vi "AlliGator All ROIs Phasor Analysis.vi"(8 "error in (no error)":errorcluster, 10 "New Plot Name":string, 11 "AlliGator Internal Variables DVR":refnum<data-value>) -> (0 "error out":errorcluster, 1 "Calibrated Phasor":T1, 2 "Phasor Plot":cluster{"g Array":dbl[], "s Array":dbl[]}, 3 "AlliGator Internal Variables DVR":refnum<data-value>, 4 "Calibrated Phase Lifetime":dbl[unit], 6 "Message":string)   [LabVIEW 2021, in "AlliGator Phasor Graph.lvlib"]
doc: "Non-interactive phasor analysis of all ROIs."
uses:
  AlliGator Phasor Graph.lvlib
  AlliGator Internal Variables v2.ctl
  <vilib>/vision/Image Controls.llb/IMAQ Image.ctl
  AlliGator Gate Image Set.ctl
  AlliGator FLI Dataset Type.ctl
  AlliGator Data Series Type.ctl
  AlliGator Dataset Channel.ctl
  AlliGator Gate Arithmetic.ctl
  AlliGator Displayed Image.ctl
  Image/Named ROI Description.ctl
  AlliGator Decay Metadata v3.ctl
  AlliGator Decay Background Subtraction Info.ctl
  AlliGator Baseline Subtraction Method.ctl
  Graphs/XY Graph/XY Graph Plot Shift Parameters.ctl
  Graphs/XY Graph/XY Graph Plot Shift Method.ctl
  AlliGator Decay Extrapolation Parameters.ctl
  Phasor/Calibration Phasor (m, phi).ctl
  Phasor/Phasor Reference Series.ctl
  Phasor/Phasor Calibration Map v2.ctl
  Phasor/Phasor (g, s).ctl
  AlliGator Raw Phasor Plot Data v4.ctl
  Phasor/Phasor Standard Deviation Options.ctl
  AlliGator Phasor Multi-Harmonic Data.ctl
  Phasor/Phasor Harmonic Data.ctl
  AlliGator Decay Fit Options & Parameters v2.ctl
  Fits/IRF(X)PSED/Decay Fit Options v2.ctl
  Fits/Decay Convolution/Decay Model.ctl
  Fits/Residual Type.ctl
  Fits/IRF(X)PSED/Fit Weights Type.ctl
  Fits/Non-linear Fitting Method v2.ctl
  Fits/Fit Calculation Method.ctl
  Fits/Non-linear Fitting Algorithm.ctl
  AlliGator Decay Fit Parameter Constraints 2.ctl
  Fits/IRF(X)PSED/Decay Fit Parameters In List.ctl
  Fits/IRF(X)PSED/MLE Baseline Offset Type.ctl
  AlliGator Decay Preprocessing Parameters.ctl
  Fits/IRF(X)PSED/Decay Fit Parameters & Derived Quantities List.ctl
  AlliGator Variables List.ctl
  AlliGator Settings List.ctl
  Variant/Variant to Data/Variant to U16.vi
  <vilib>/Utility/error.llb/Error Cluster From Error Code.vi
  AlliGator Abort.vi
  <vilib>/ErrorRing/Error Ring.xnode
  AlliGator Globals, Variables & Constants.lvlib
  Image/Image.lvlib
  AlliGator Decay Processing.lvlib
  AlliGator Source Image.lvlib
  AlliGator Phasor Calibration.lvlib
  AlliGator Settings.lvlib
  Phasor/Phasor.lvlib
  Strings/Strings.lvlib
  Time/Time.lvlib
  AlliGator Decay Preprocessing.lvlib
  Graphs/XY Graph/XY Graph Add-Ons.lvlib
  GUI/GUI.lvlib
  Notebook/Notebook.lvlib
  Rich Text Box/Rich Text Box.lvlib
  Error/Error.lvlib
  Variant/Variant to Data/Variant to Data.lvlib
  AlliGator Files.lvlib
  AlliGator Internal Variables.lvlib
  AlliGator Phasor Plot.lvlib
  Fits/Fits.lvlib
  AlliGator Decay Fit.lvlib
  AlliGator Decay Fit Parameter Map.lvlib
  AlliGator Dual-Channel Datasets.lvlib
panel:
  # "see the AlliGator License on the block diagram (Ctrl+E or Window:Show Block Diagram)"
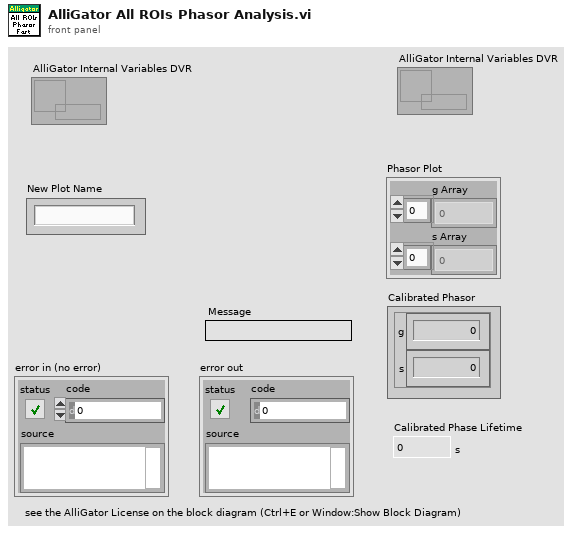
[diagram p1: front panel]
types:
  T1 = typedef "Phasor.lvlib/Phasor (g, s).ctl" = cluster{"g":dbl, "s":dbl}
  T2 = typedef "Phasor.lvlib/Phasor Standard Deviation Options.ctl" = cluster{"Compute Estimated SDV":bool, "# Replicas":u32, "Use Estimated Average Phasor":bool}
  T3 = typedef "AlliGator Settings.lvlib/AlliGator Settings List.ctl" = enum16{"GUI:Visible Settings Tab", "GUI:Last Run Version", "Source Image:Use Image Histogram for Contrast", "Source Image:Low Count Pixels Rejection Options", "Source Image:High Count Pixels Rejection Options", "Source Image:Use Image Brightness", "Source Image:Blend Overlay with Image Background", "Source Image:Use Fixed ROI Diameter", "Source Image:ROI Diameter", "Source Image:ROI Center Color", "Source Image:Peak Threshold", "Source Image:Intensity Threshold", "Source Image:Image Binning Options", "Source Image:Image Smoothing Options", "Source Image:Image Histogram Active", "Source Image:Invert Binary Mask", "Source Image:Hot Pixel Removal", "Source Image:Overlay Analyzed ROI Center", "Source Image:Auto-Adjust Contrast", "Source Image:Histogram Lower Percentile", "Source Image:Histogram Upper Percentile", "Source Image:Save Source Image", "Source Image:Scale Bar Options", "Source Image:Image Resolution (Pixel Size)", "Source Image:Flatfield Correction", "Source Image:Show Dead Left Columns Correction", "Source Image:Dead Left Columns Correction", "Source Image:Image Pre-Processing Operations Order", "Data Information:Gate Width", "Data Information:Nanotime Gate Separation", "Data Information:Macrotime Gate Separation", "Data Information:Gate Step", "Data Information:# Gates", "Data Information:Gate Image Exposure", "Data Information:Gate Image Integration", "Data Information:Gates to Skip", "Data Information:Gates to Keep", "Data Information:Define Gates to", "Data Information:Channel Name", "Data Information:Available Channel Names", "Data Information:Channel Arithmetic", "Data Information:Background File Subtraction", "Data Information:Background File", "Data Information:Background Scaling Factor", "Data Information:Background Pile-up Correction", "Data Information:Background Pixel Well Capacity", "Data Information:Laser Period", "Data Information:SYNC Period", "Data Information:Pile-up Correction", "Data Information:Pixel Well Capacity", "Data Information:Dataset Scaling Factor", "Fluorescence Decay_Decay Pre-Processing:Reverse Gates", "Fluorescence Decay_Decay Pre-Processing:Verbose Decay Pre-Processing", "Fluorescence Decay_Decay Pre-Processing:Use Decay Pre-Processing", "Fluorescence Decay_Decay Pre-Processing:Background Subtraction", "Fluorescence Decay_Decay Pre-Processing:Background Definition Range", "Fluorescence Decay_Decay Pre-Processing:Baseline Subtraction Method", "Fluorescence Decay_Decay Pre-Processing:Decay Pre-Processing Operations Order", "Fluorescence Decay_Decay Pre-Processing:Smoothing Parameter", "Fluorescence Decay_Decay Pre-Processing:Shift Decay", "Fluorescence Decay_Decay Pre-Processing:Decay Shift Parameters", "Fluorescence Decay_Decay Pre-Processing:Fold Decay", "Fluorescence Decay_Decay Pre-Processing:# Folds", "Fluorescence Decay_Decay Pre-Processing:1-Normalize Decay", "Fluorescence Decay_Decay Pre-Processing:[0-1]-Normalize Decay", "Fluorescence Decay_Decay Pre-Processing:Smoothen Decay", "Fluorescence Decay_Decay Pre-Processing:Extrapolate Decay", "Fluorescence Decay_Decay Pre-Processing:Use Periodicity", "Fluorescence Decay_Decay Pre-Processing:Use Cursors", "Fluorescence Decay_Decay Pre-Processing:Tail Fraction", "Fluorescence Decay_Decay Pre-Processing:Head Fraction", "Fluorescence Decay_Decay Pre-Processing:Additional Points", "Fluorescence Decay_Decay Pre-Processing:Straighten Decay", "Fluorescence Decay_Decay Pre-Processing:Constant Background", "Fluorescence Decay_Decay Pre-Processing:Pixel-Normalize Decay", "Fluorescence Decay_Advanced Analysis:Extract IRF instead of Decay", "Fluorescence Decay_Advanced Analysis:IRF Extraction Options", "Fluorescence Decay_Advanced Analysis:IRF Optimization Options", "Fluorescence Decay_Advanced Analysis:Square Pulse Options", "Fluorescence Decay_Advanced Analysis:IRF Order", "Fluorescence Decay_Advanced Analysis:IRF Time Constants", "Fluorescence Decay_Advanced Analysis:Wavelet Analysis Options", "Fluorescence Decay_Advanced Analysis:Average Lifetime Options", "Fluorescence Decay_Fit Options:Fit Options", "Fluorescence Decay_Fit Options:Use Legacy Fitting Approach", "Fluorescence Decay_Fit Options:Use Data Information Laser Period", "Fluorescence Decay_Fit Parameters:Displayed Fit Parameters", "Fluorescence Decay_Fit Parameters:Fit Parameter Constraints", "Fluorescence Decay_Fit Parameters:Export Tabulated Results", "Fluorescence Decay_Fit Parameters:MLE Baseline Offset Type", "Fluorescence Decay_Fit Parameters:MLE Baseline Offset", "Fluorescence Decay_Fit Parameters:Guess Parameter Names", "Fluorescence Decay_Fit Parameters:Guess Parameter Values", "Fluorescence Decay_Fit Parameters:Guess Parameters Options", "Fluorescence Decay_Styles:Show Last Decay Only", "Fluorescence Decay_Styles:Decay Graph Color Array", "Fluorescence Decay:Decay Graph Active", "Fluorescence Decay Statistics:Min Peak Value", "Fluorescence Decay Statistics:Reject Low Decay Peak Pixels", "Fluorescence Decay Statistics:Reject High Decay Peak Pixels", "Fluorescence Decay Statistics:Max Peak Value", "Time Traces:Use File Timestamp", "Time Traces:Time Step", "Time Traces:Use Intensity Correction File", "Time Traces:Intensity Correction File", "Phasor Plot:Phasor Plot Smoothing Options", "Phasor Plot:Phasor Plot Size", "Phasor Plot:Phasor Plot Graphics Options", "Phasor Plot:Cumulative Phasor Plot", "Phasor Plot:Use Phasor Brightness", "Phasor Plot:Blend Overlay with Phasor Background", "Phasor Plot:Save Phasor Plot", "Phasor Plot:Show References", "Phasor Plot:Phasor Ratio Decay Range", "Phasor Plot:Exponential Fading", "Phasor Plot:Phasor Ratio Reference Colors", "Phasor Plot:Reference Radius", "Phasor Plot:Show Color Map Vertices", "Phasor Plot:Phasor Plot Active", "Phasor Plot:Phasor Ratio Color Map Type", "Phasor Plot:Phasor Ratio Color Map", "Phasor Plot:Phasor Ratio Display Range", "Phasor Plot:Selected Image ROI(s)", "Phasor Plot:All Image ROIs", "Phasor Plot:Selected Phasor Plot ROI(s)", "Phasor Plot:All Phasor Plot ROIs", "Phasor Plot:Phasor Ratio Color-Coded Quantity", "Phasor Plot:Store Phasor Harmonics", "Phasor Plot:Draw Reference Segment", "Phasor Plot:User-Defined Quantity", "Phasor Graph:Phasor Frequency", "Phasor Graph:Phasor Ratio Type", "Phasor Graph:Pixel-level Phasor Computation", "Phasor Graph:Save Phasor Graph", "Phasor Graph:Phasor Graph Active", "Phasor Graph:Phasor SDV Options", "Phasor Calibration:Use Backup Calibration if needed", "Phasor Graph:Define Shortest Lifetime as", "Phasor Calibration:Backup Calibration Type", "Phasor Calibration:Calibration Type", "Phasor Calibration:Calibration Lifetime", "Phasor Calibration:Calibration Map Algorithm", "Single-Exponential Phasor Locus (SEPL):Gate Parameters", "Single-Exponential Phasor Locus (SEPL):User-defined Gate", "Single-Exponential Phasor Locus (SEPL):User-defined IRF", "Single-Exponential Phasor Locus (SEPL):Phasor Parameters", "Single-Exponential Phasor Locus (SEPL):Decay & IRF Parameters", "Single-Exponential Phasor Locus (SEPL):Display Parameters", "Lifetime Analysis:Decay Analysis Parameters", "Lifetime Analysis:Lifetime Map Active", "Plugins:Python Settings", "Miscellaneous:Verbose Mode", "Miscellaneous:Beep after Script", "Miscellaneous:Saved Image File Format", "Miscellaneous:Exported Gate Image Settings", "Miscellaneous:Include Loading in Timing", "Miscellaneous:Verbose Settings Mode", "Miscellaneous:Histogram Options", "Miscellaneous:Beep on Error", "Miscellaneous:# Logical Processors Used", "Miscellaneous:ROI Description Max Characters", "Miscellaneous:Verbose Error Mode", "Miscellaneous:Transparent Mask Color"}
  T4 = typedef "AlliGator Globals, Variables & Constants.lvlib/AlliGator Variables List.ctl" = enum16{"---- GUI ----", "Initialization Status", "State Indicators Refnum", "Original AlliGator Menu Items", "Current Action Loop State", "Script in progress", "Playback", "Loop Playback", "Search ROI Used", "Search ROI", "Decay Graph Max Legend Size", "Intensity Graph Max Legend Size", "Decay Statistics Graph Max Legend Size", "Phasor Graph Max Legend Size", "Phasor Ratio Graph Max Legend Size", "Lifetime Graph Max Legend Size", "---- Files ----", "Export Dataset Frames as Individual Files", "Show Batch Export Help Balloons", "Frames in Dataset", "ptu File Frame Start Indices", "Current Frame in Dataset", "Current Frame Timestamp", "------ Python Plugins ------", "Python Plugins Information", "Python Session", "Valid Python Session?", "---- Source Image ----", "Dataset Loaded", "Dataset Metadata", "Dataset Channel", "Dataset Data Description", "Background Dataset Metadata", "Background Dataset Channel", "Background Dataset Data Description", "Background File Subtraction", "Background File Path", "Background File Pile-up Correction", "Background File Pixel Well Capacity", "Background File Scaling Factor", "Source Image ROIs", "Current Source Image ROI", "Source Image ROI Event Refnum", "X_Source Image Display Range", "X_Source Image Palette Information", "Source Image Palette List", "Source Image Scale", "Current Dataset Load Settings", "Source Image:ROI Overlay Color", "---- Image Profile Window ----", "Image Profile:Overlay ROI in Source Image", "Image Profile Window Event Refnum", "Image Profile:IntensityType", "Image Profile:Intensity Average Type", "Image Profile:Intensity-weighted SDV", "Image Profile:Box Profile Type", "Image Profile Window Open", "Image Profile:Plotted Fit Parameter", "X_Type of Displayed Image", "X_Time Gate Slider", "Dataset Path", "Source Image Overlay to Erase", "Is Displayed Image Accumulated", "White Light Image Modified", "Mask Image Modified", "Macrotime Gate Separation", "------ Phasor Graph -------", "Phasor Graph:Show Line", "---- Phasor Plot ---", "Phasor Plot Parameters Changed", "FLI Dataset Modified since last Phasor Plot Calculation", "Phasor Harmonics Data", "Selected Phasor Harmonics", "Phasor Harmonic Manager Event Refnum", "Phasor Plot ROIs", "Current Phasor Plot ROI", "Phasor Plot ROI Event Refnum", "Phasor Plot Image Reference Points", "Phasor Plot Computed", "Phasor Plot Palette Information", "Phasor Plot Palette List", "Phasor Ratio Palette Information", "Phasor Ratio Palette List", "Phasor Image Scale", "Phasor Plot Image Overlay to Erase", "Phasor Plot Image Elements to Update", "Current Phasor Plot Calculation Parameters", "Current Phasor Calibration Options", "Reset Cumulated Phasor Plot", "Phasor Ratio Reference 1", "Phasor Ratio Lifetime Reference 1", "Phasor Ratio Reference 1 Frequency", "Phasor Ratio Reference 2", "Phasor Ratio Lifetime Reference 2", "Phasor Ratio Reference 2 Frequency", "---- Decay Analysis ----", "Number of Selected Decays to Fit", "LS Fit Results", "LAR Fit Results", "BS Fit Results", "Last Decay Max - Min", "Best Fit Parameters", "Best Fit Parameter Names", "Actual Size X", "Actual Size Y", "Binning X", "Binning Y", "Actual # Gates", "Dataset Number", "Gates to...", "Gates Skipped", "Gates to keep", "Gate Step", "Gate Separation", "Reversed Gates", "Pile-up Correction", "Pixel Well Capacity", "Background Subtracted", "Background Subtraction Method", "Background Definition Range", "Background File (deprecated)", "Number of Dataset Accumulated", "Array of Accumulated Dataset Paths", "Do Averaged Datasets", "Destination File Path", "Process Plot Target", "Use 1/D as Phasor Frequency", "---- Decay Fit Parameter Map -----", "Decay Fit Parameter Map Palette Information", "Decay Fit Parameter Map Palette List", "Local Decay Graph Window Event Refnum", "------- Local Decay Window ---------", "Use normalized IRF for convolution", "----- Miscellaneous ----", "Skippable Dialog Windows Status"}
  T5 = typedef "IMAQ Image.ctl" = refnum<image>
  T6 = typedef "Image.lvlib/Named ROI Description.ctl" = cluster{"ROI Descriptor":T7, "ROI Name":string, "Overlay Color":u32}
  T7 = typedef "ROI Descriptor" = cluster{"Global Rectangle":i32[], "Contours":cluster{"ID":enum32{"External", "Internal"}, "Type":u32, "Coordinates":i32[]}[]}
  T8 = typedef "AlliGator Phasor Graph.lvlib/AlliGator Raw Phasor Plot Data v4.ctl" = cluster{"Phasor Plot Name":string, "Raw Phasor Plot":T1[], "Phasor Frequency":dbl[unit], "[Decay Metadata]":T9[], "Raw Phasor Plot SDV":T1[], "Phasor SDV Options":T2, "[Calibration Phasor]":T15[]}
  T9 = typedef "AlliGator Phasor Graph.lvlib/AlliGator Decay Metadata v3.ctl" = cluster{"ROI Descriptor":T7, "ROI Center":cluster{"X":i32, "Y":i32}, "Decay Background Subtraction Info":T10, "Decay Reverted":bool, "Decay Smoothened":bool, "Decay Straightened":bool, "Fitted Tau (Decay Straightening)":dbl, "Decay Shift Parameters":T12, "Decay Shifted":bool, "Decay Extrapolated":bool, "Decay Extrapolation Parameters":T14, "Decay Normalized":bool, "Fold Decay":bool, "# Folds":u32}
  T10 = typedef "AlliGator Decay Analysis.lvlib/AlliGator Decay Preprocessing.lvlib/AlliGator Decay Background Subtraction Info.ctl" = cluster{"Laser Period":dbl[unit], "Gate Duration":dbl[unit], "Baseline Subtraction Method":T11, "Background Definition Range":cluster{"Min Gate":dbl[unit], "Max Gate":dbl[unit]}, "Total Intensity w/o Bkgd Subtraction":dbl, "Bkgd-subtracted Intensity (exp)":dbl, "# Data Points":i32, "Background/Gate":dbl, "Fitted Lifetime":dbl[unit], "Bkgd-subtracted Intensity (theo)":dbl}
  T11 = typedef "AlliGator Decay Analysis.lvlib/AlliGator Decay Preprocessing.lvlib/AlliGator Baseline Subtraction Method.ctl" = enum16{"Mean", "Min", "Square Gated Single-Exponential", "File", "Constant"}
  T12 = typedef "XY Graph Add-Ons.lvlib/XY Graph Plot Shift Parameters.ctl" = cluster{"Type":T13, "Shift":dbl[unit], "Threshold":dbl, "Rotate":bool}
  T13 = typedef "XY Graph Add-Ons.lvlib/XY Graph Plot Shift Method.ctl" = enum16{"Default", "CFD", "Threshold", "Cross-Correlation"}
  T14 = typedef "AlliGator Decay Analysis.lvlib/AlliGator Decay Preprocessing.lvlib/AlliGator Decay Extrapolation Parameters.ctl" = cluster{"Additional Points":u32, "Head Fraction":dbl, "Fitted Tau":dbl, "Use Periodicity":bool, "Use Cursors":bool, "Tail Fraction":dbl}
  T15 = typedef "Phasor.lvlib/Calibration Phasor (m, phi).ctl" = cluster{"m":dbl, "phi":dbl, "Phasor Frequency":dbl[unit], "Reference Lifetime":dbl[unit]}
  T16 = typedef "AlliGator Internal Variables.lvlib/AlliGator Internal Variables v2.ctl" = cluster{"Displayed Image":T5, "White Light Image":T5, "Mask Image":T5, "ROI Mask Image":T5, "Current Dataset Images 1":T17, "Background Dataset Images 1":T17, "Current Dataset Images 2":T17, "Background Dataset Images 2":T17, "Current Dataset Arithmetic Images":T17, "Accumulated Dataset Images 1":T17, "Accumulated Dataset Images 2":T17, "Accumulated Dataset Arithmetic Images":T17, "Phasor Plot Image":T5, "Decay Fit Parameter Map Image":T5, "Single Data Point Path":path, "White Light Image Path":path, "Mask Image Path":path, "Time-Series Folder":path, "[Time-Series Paths]":path[], "Current Dataset":i32, "Single Dataset Type":T18, "Current Folder":string, "AlliGator Data Series Type":T19, "# Datasets":i32, "Dual-Channel Dataset":bool, "Selected Channel Name":string, "Dataset Channel":T20, "Channel Arithmetic":T21, "Dual-Channel Background Dataset":bool, "Background Channel":T20, "Dual-Channel Accumulated Dataset":bool, "Start Time":dbl, "[Time-Series Timestamps]":dbl[], "[Intensity Corrections]":dbl[], "Time Series Script":bool, "Type of Displayed Image":T22, "Gate Image Slide":u16, "# Gates":i32, "ROIs":T6[], "ROI Decay":cluster{"t Array":dbl[], "I Array":dbl[]}, "Valid Decay":bool, "Decay  Metadata":T9, "Reference Decay Plot Name":string, "Reference Decay":cluster{"t Array":dbl[], "I Array":dbl[]}, "Decay Shift Plot":cluster{"Time Stamps":dbl[], "Decay Shifts":dbl[]}, "[Decays Max Values]":sgl[], "[Decays Min Values]":sgl[], "Calibration Phasor":T15, "Calibration Phasor Series":T23, "Phasor Calibration Map":T24, "Calibration Map MD5 Digest":string, "Last Raw Phasor":T1, "Last Calibrated Phasor":T1, "Last Calibrated Phasor SDV":T1, "Phasor Graph:Phasor Plot":cluster{"g Array":dbl[], "s Array":dbl[]}, "Phasor Graph:Phasor SDV Plot":cluster{"g Array":dbl[], "s Array":dbl[]}, "[Phasor Graph:Raw Phasor Plots]":T8[], "Phasor Plot locked to Ref 1":i32, "[Phasor Plot(s) locked to Ref 1]":i32[], "[Phasor Plot(s) locked to Ref 2]":i32[], "[Pixel Phasors]":T1[], "[[Sum Image]]":dbl[][], "[[CSG Phasors]]":csg[][], "[[Valid Pixel?]]":bool[][], "I/m/phi Dataset":cluster{"I/m/phi Dataset?":bool, "Base Frequency":dbl[unit], "Harmonic Orders":u8[]}, "Multi Phasor Plot Data":T25, "Decay Fit Options & Parameters":T27, "Fit Options: Decay Preprocessing Parameters":T38, "Fit Options: Reference Decay":cluster{"t Array":dbl[], "I Array":dbl[]}, "Is Full Image Parameters Map":bool, "Is Single-Pixels Parameters Map":bool, "NLSF Parameters Map X Resolution":i32, "NLSF Parameters Map Y Resolution":i32, "[Single Decay Fit Parameters]":dbl[], "Fit Model":T29, "[[Multiple Decays Fit Parameters]]":dbl[][], "[[Multiple Decays Fit Parameter SDVs]]":dbl[][], "[[IRFs]]":dbl[][], "IRF Array Time Axis":dbl[], "Decay Array Time Axis":dbl[], "[Decay Fit Parameter Names]":T39[], "[[Phasor Ratios]]":dbl[][], "[[Average Lifetimes]]":dbl[][], "Amplitude Weighted Average Lifetime":bool, "[Decay Sum]":dbl[], "[[User-defined Quantities]]":dbl[][], "User-defined Quantity":string}
  T17 = typedef "AlliGator Internal Variables.lvlib/AlliGator Gate Image Set.ctl" = cluster{"SGL Image Max":T5, "SGL Image Sum":T5, "SGL Gate Images":T5[], "SGL Image Min":T5}
  T18 = typedef "AlliGator Files.lvlib/AlliGator FLI Dataset Type.ctl" = enum16{"HDF5 FLI Dataset", "Gate Image Folder", ".sdt FLI Dataset (Becker & Hickl)", ".ptu FLI Dataset (PicoQuant)", "SS1 FLI Dataset", "SS2 FLI Dataset", "I/m/phi Dataset", ".bin FLI Dataset (PicoQuant Binned)", ".bin FLI Dataset (Piccolo Binned)"}
  T19 = typedef "AlliGator Files.lvlib/AlliGator Data Series Type.ctl" = enum16{"Not a Supported Series", "Gate Images Folder Series", "SwissSPAD 2 Dataset Series", "B&H FLI Dataset Series", "PicoQuant PTU FLI Dataset Series", "PicoQuant BIN FLI Dataset Series", "Piccolo hist BIN FLI Dataset Series", "HDF5 FLI Dataset Series"}
  T20 = typedef "AlliGator Dual-Channel Datasets.lvlib/AlliGator Dataset Channel.ctl" = enum16{"G2", "INT"}
  T21 = typedef "AlliGator Settings.lvlib/AlliGator Gate Arithmetic.ctl" = enum16{"None", "INT-G2", "G2/INT*<INT>", "(1 - G2/INT)*<INT>"}
  T22 = typedef "AlliGator Source Image.lvlib/AlliGator Displayed Image.ctl" = enum16{"Single Gate", "Sum of All Gates", "Max of All Gates", "Min of All Gates", "-", "White Ligth Image", "Mask Image"}
  T23 = typedef "Phasor.lvlib/Phasor Reference Series.ctl" = cluster{"m Array":dbl[], "phi Array":dbl[], "Phasor Frequency":dbl[unit], "Calibration Lifetime":dbl[unit]}
  T24 = typedef "Phasor.lvlib/Phasor Calibration Map v2.ctl" = cluster{"Phasor Frequency":dbl[unit], "Calibration Lifetime":dbl[unit], "ROI Centers":cluster{"X":i32, "Y":i32}[], "ROI Descriptors":T7[], "Map Resolution X":i32, "Map Resolution Y":i32, "z Array":cdb[]}
  T25 = typedef "AlliGator Phasor Plot.lvlib/AlliGator Phasor Multi-Harmonic Data.ctl" = cluster{"Base Frequency":dbl[unit], "# Harmonics":u8, "Harmonic Orders":u8[], "Phasor Plot Settings Checksum":u64, "Phasor Harmonic Data Array":T26[]}
  T26 = typedef "Phasor.lvlib/Phasor Harmonic Data.ctl" = cluster{"Phasor Harmonic Name":string, "Phasor Plot Settings Checksum":u64, "Phasor Frequency":dbl[unit], "Base Frequency":dbl[unit], "Harmonic Order":u8, "Phasor Plot Parameters":string, "Phasor Array [[CSG]]":csg[][], "Dataset File Path":path}
  T27 = typedef "AlliGator Decay Fit Parameter Map.lvlib/AlliGator Decay Fit Options & Parameters v2.ctl" = cluster{"SYNC Period":dbl[unit], "Fit Options":T28, "Fit Parameter Constraints":T35[], "MLE Baseline Offset":dbl, "MLE Baseline Offset Type":T37}
  T28 = typedef "Fits.lvlib/Decay Fit Options v2.ctl" = cluster{"Show Fit Residuals":bool, "Fit Model":T29, "Residual Type":T30, "Max Decay Percentile":dbl, "Min Decay Percentile":dbl, "Show Full Decay":bool, "Weights":T31, "Fitting Method":T32, "Compute Parameter Uncertainties":bool, "Periodic Boundaries":bool, "Model Calculation":T33, "Period":dbl[unit], "Termination Criteria":cluster{"Max Iterations":i32, "Max Function Calls":i32, "Max Time":dbl[unit], "Function Tolerance":dbl, "Parameter Tolerance":dbl, "Gradient Tolerance":dbl, "Min Lambda":dbl, "Max Lambda":dbl, "Initial Tick Count":u32}, "Offset Resolution":dbl[unit], "Use Local IRF":bool, "Fitting Algorithm":T34}
  T29 = typedef "Fits.lvlib/Decay Model.ctl" = enum16{"1-Exponential", "2-Exponentials"}
  T30 = typedef "Fits.lvlib/Residual Type.ctl" = enum16{"Standard", "Normalized", "Reduced"}
  T31 = typedef "Fits.lvlib/Fit Weights Type.ctl" = enum16{"Unweighted", "1/Variance", "Best of All"}
  T32 = typedef "Fits.lvlib/Non-linear Fitting Method v2.ctl" = enum16{"Least Square", "Least Absolute Residual", "Bisquare", "MLE", "-", "Best of All"}
  T33 = typedef "Fits.lvlib/Fit Calculation Method.ctl" = enum16{"Simulation", "Convolution", "Integration"}
  T34 = typedef "Fits.lvlib/Non-linear Fitting Algorithm.ctl" = enum16{"Levenberg-Marquardt", "Trust-Region Dogleg"}
  T35 = typedef "AlliGator Decay Analysis.lvlib/AlliGator Decay Fit.lvlib/AlliGator Decay Fit Parameter Constraints 2.ctl" = cluster{"Fit Parameter":T36, "Min Value":dbl, "Max Value":dbl, "Global":bool, "Used":bool}
  T36 = typedef "Fits.lvlib/Decay Fit Parameters In List.ctl" = enum16{"Offset", "Baseline", "A_1", "tau_1", "A_2", "tau_2"}
  T37 = typedef "Fits.lvlib/MLE Baseline Offset Type.ctl" = enum32{"Absolute", "Percentage"}
  T38 = typedef "AlliGator Decay Analysis.lvlib/AlliGator Decay Preprocessing.lvlib/AlliGator Decay Preprocessing Parameters.ctl" = cluster{"Background Subtraction":bool, "Straighten Decay":bool, "Reverse Gates":bool, "1-Normalized Decay":bool, "Smoothen Decay":bool, "Smoothing Parameter":dbl, "Shift Decay":bool, "Decay Shift Parameters":T12, "Extrapolate Decay":bool, "Additional Points":u32, "Head Fraction":dbl, "Pixel-Normalize Decay":bool, "Use Periodicity":bool, "Use Cursors":bool, "Tail Fraction":dbl, "Use Decay Pre-Processing":bool, "Fold Decay":bool, "# Folds":u32, "[0-1]-Normalized Decay":bool}
  T39 = typedef "Fits.lvlib/Decay Fit Parameters & Derived Quantities List.ctl" = enum16{"Offset", "Baseline", "A_1", "tau_1", "A_2", "tau_2", "<tau>_a", "f1_a", "f2_a", "<tau>_i", "f1_i", "f2_i", "-", "R^2", "Chi^2"}
  T40 = cluster{"Decay Peak Constraint":bool, "Min":dbl, "Max":dbl}
  T41 = typedef "AlliGator Settings.lvlib/AlliGator Pixel Counts Constraints.ctl" = cluster{"High Count Pixels Rejection Options":T42, "Low Count Pixels Rejection Options":T43}
  T42 = typedef "AlliGator Settings.lvlib/AlliGator High Count Pixels Rejection Options.ctl" = cluster{"Background High Threshold Factor":dbl, "Fixed High Background Threshold":dbl, "Reject High Count Pixels":bool, "High Percentile":dbl}
  T43 = typedef "AlliGator Settings.lvlib/AlliGator Low Count Pixels Rejection Options.ctl" = cluster{"Background Low Threshold Factor":dbl, "Fixed Low Background Threshold":dbl, "Reject Low Count Pixels":bool, "Low Percentile":dbl}
  T44 = cluster{"t Axis":dbl[], "ROI Intensity Array":dbl[]}
  T45 = typedef "Rich Text Box.lvlib/Text Formatting.ctl" = cluster{"Font":string, "Text Color":T46, "Text Background Color":T46, "Text Style":enum16{"Regular", "Bold", "Italic", "Underline", "Strikeout"}, "Font Size (Points)":dbl, "Text Alignment":i32}
  T46 = typedef "Rich Text Box.lvlib/Text Colors.ctl" = enum16{"Unchanged", "Black", "Blue", "Brown", "Gray", "Green", "Orange", "Pink", "Red", "White"}
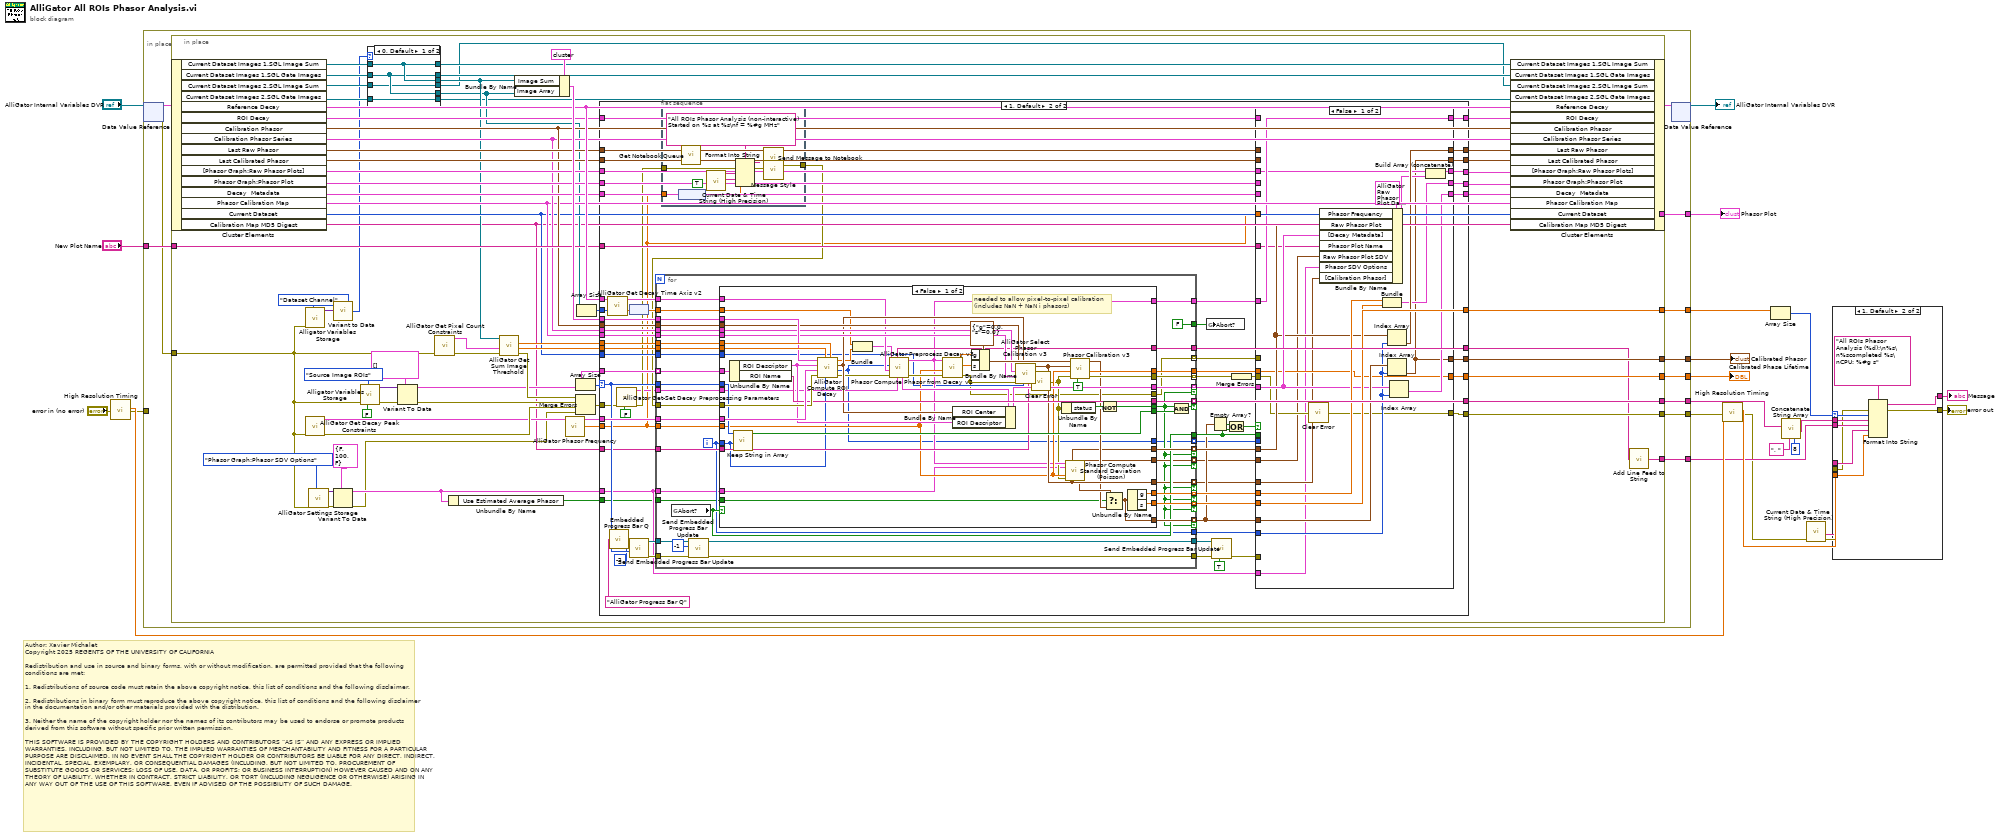
[diagram p0: block diagram]
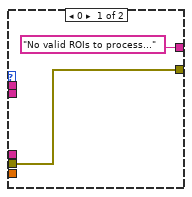
[diagram p2: hidden frame]
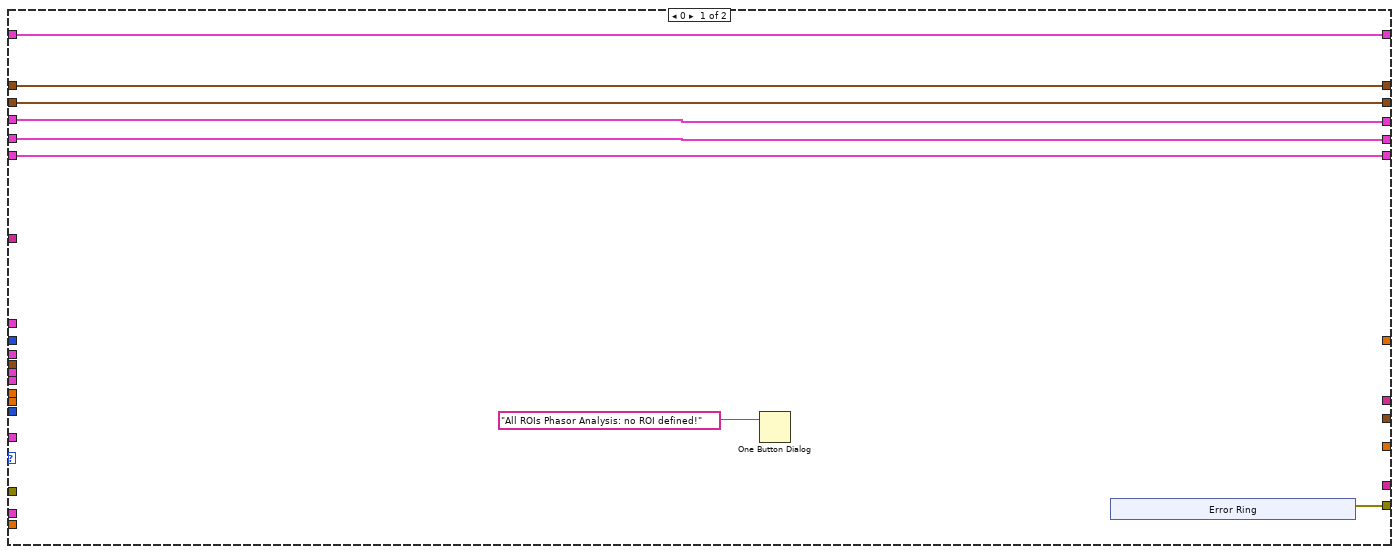
[diagram p4: hidden frame]
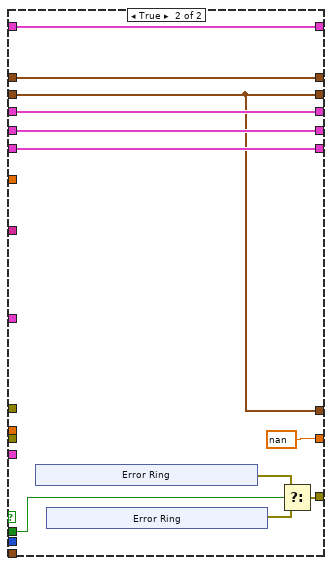
[diagram p5: hidden frame]
diagram:
  # "Author: Xavier Michalet\nCopyright 2025 REGENTS OF THE UNIVERSITY OF CALIFORNIA\n\nRedistribution and use in source and binary forms, with or without modification, are permitted provided that the following conditions are met:\n\n1. Redistributions of source code must retain the above copyright notice, this list of conditions and the following disclaimer.\n\n2. Redistributions in binary form must reproduce the above copyright notice, this list of conditions and the following disclaimer in the documentation and/or other materials provided with the distribution.\n\n3. Neither the name of the copyright holder nor the names of its contributors may be used to endorse or promote products derived from this software without specific prior written permission.\n\nTHIS SOFTWARE IS PROVIDED BY THE COPYRIGHT HOLDERS AND CONTRIBUTORS “AS IS” AND ANY EXPRESS OR IMPLIED WARRANTIES, INCLUDING, BUT NOT LIMITED TO, THE IMPLIED WARRANTIES OF MERCHANTABILITY AND FITNESS FOR A PARTICULAR PURPOSE ARE DISCLAIMED. IN NO EVENT SHALL THE COPYRIGHT HOLDER OR CONTRIBUTORS BE LIABLE FOR ANY DIRECT, INDIRECT, INCIDENTAL, SPECIAL, EXEMPLARY, OR CONSEQUENTIAL DAMAGES (INCLUDING, BUT NOT LIMITED TO, PROCUREMENT OF SUBSTITUTE GOODS OR SERVICES; LOSS OF USE, DATA, OR PROFITS; OR BUSINESS INTERRUPTION) HOWEVER CAUSED AND ON ANY THEORY OF LIABILITY, WHETHER IN CONTRACT, STRICT LIABILITY, OR TORT (INCLUDING NEGLIGENCE OR OTHERWISE) ARISING IN ANY WAY OUT OF THE USE OF THIS SOFTWARE, EVEN IF ADVISED OF THE POSSIBILITY OF SUCH DAMAGE."
  n1 = call "High Resolution Timing.vi"("Error In"="error in (no error)") -> ("elapsed (relative) seconds"=w13:dbl, "Error Out"=w7:errorcluster)  [unwired: 16 in, 1 out]
  n2 = in-place {
    in-place-border: [w32] -> w4
    in-place-border: [w31] -> w20
    in-place-border: "New Plot Name" -> [w30]
    in-place-border: [w29] -> w18
    in-place-border: [w28] -> w17
    in-place-border: [w27] -> w9
    in-place-border: w7 -> [_]
    in-place-border: [w25] -> w6
    in-place-border: [w24] -> w3
    n3 = in-place-dvr #1("AlliGator Internal Variables DVR") -> (w34:T16, w26:errorcluster)
    n4 = in-place {
      in-place-border: w26 -> [w43]
      in-place-border: [w85] -> w32
      in-place-border: [w73] -> w31
      in-place-border: w30 -> [w72]
      in-place-border: [w71] -> w29
      in-place-border: [w70] -> w28
      in-place-border: [w69] -> w27
      in-place-border: [w67] -> w25
      in-place-border: [w59] -> w24
      n5 = in-place-cluster #2(w34) -> ("Current Dataset Images 1.SGL Image Sum"=w53:T5, "Current Dataset Images 1.SGL Gate Images"=w52:T5[], "Current Dataset Images 2.SGL Image Sum"=w56:T5, "Current Dataset Images 2.SGL Gate Images"=w55:T5[], "Reference Decay"=w86:cluster{"t Array":dbl[], "I Array":dbl[]}, "ROI Decay"=w75:cluster{"t Array":dbl[], "I Array":dbl[]}, "Calibration Phasor"=w66:T15, "Calibration Phasor Series"=w65:T23, "Last Raw Phasor"=w84:T1, "Last Calibrated Phasor"=w82:T1, "[Phasor Graph:Raw Phasor Plots]"=w80:T8[], "Phasor Graph:Phasor Plot"=w78:cluster{"g Array":dbl[], "s Array":dbl[]}, "Decay  Metadata"=w77:T9, "Phasor Calibration Map"=w64:T24, "Current Dataset"=w62:i32, "Calibration Map MD5 Digest"=w51:string)
      n6 = call "Alligator Variables Storage.vi"("AlliGator Variable"=AlliGator_Variables_List."Dataset Channel" ("Alligator Variable"), "Error In"=w43) -> ("Data out"=w49:variant)  [unwired: 7 in, 2 out]
      n7 = call "AlliGator Get Decay Peak Constraints.vi"("error in (no error)"=w43) -> ("Error Out"=w90:errorcluster, "Decay Peak Constraints"=w89:T40)  [unwired: 9 in]
      n8 = call "AlliGator Settings Storage.vi"("AlliGator Settings List"=AlliGator_Settings_List."Phasor Graph:Phasor SDV Options", "Error In"=w43) -> ("Error Out"=w47:errorcluster, "Variant Data out"=w46:variant)  [unwired: 8 in]
      n9 = call-poly "Variant to Data.vi"("Variant"=w49) -> ("U16 Value"=w48:u16)  [unwired: 8 in]
      n10 = Variant To Data(error in=w47, type=T2 {"Compute Estimated SDV"=FALSE, "# Replicas"=100, "Use Estimated Average Phasor"=FALSE} ("Phasor SDV Options"), Variant=w46) -> (data=w36:T2, error out=w35:errorcluster)
      n11 = call "Alligator Variables Storage.vi"("Get(F)/Set"=FALSE, "AlliGator Variable"=AlliGator_Variables_List."Source Image ROIs" ("Alligator Variable"), "Error In"=w43) -> ("Error Out"=w99:errorcluster, "Data out"=w100:variant)  [unwired: 6 in, 1 out]
      n12 = case shown="0, Default" w48 {
        tunnel: [w105 w107] -> w57
        tunnel: w56 -> [w103 w107]
        tunnel: [w104 w106] -> w54
        tunnel: w55 -> [w102 w106]
        tunnel: w53 -> [w105 w109]
        tunnel: w52 -> [w104 w108]
        tunnel: [w105 w109] -> w41
        tunnel: [w104 w108] -> w40
        tunnel: [w103 w107] -> w39
        tunnel: [w102 w106] -> w38
        frame 0, Default {
        }
        frame 1 {
        }
      }
      n13 = Variant To Data(error in=w99, type=T6[] [] ("Stored ROIs in"), Variant=w100) -> (data=w61:T6[], error out=w94:errorcluster)
      n14 = call "AlliGator Get Pixel Count Constraints.vi"("error in (no error)"=w43) -> ("error out"=w95:errorcluster, "Pixel Count Constraints"=w96:T41)  [unwired: 9 in]
      n15 = Unbundle By Name(w36) -> ("Use Estimated Average Phasor"=w37:bool)
      n16 = call "AlliGator Get Sum Image Threshold.vi"("error in (no error)"=w95, "Pixel Counts Constraints"=w96, "Image in"=w57) -> ("error out"=w63:errorcluster, "Pixel Threshold Low"=w91:sgl, "Pixel Threshold High"=w92:sgl)  [unwired: 2 in, 4 out]
      n17 = Bundle By Name(cluster=cluster{"Image Sum":T5, "Image Array":T5[]} {"Image Sum"=refnum, "Image Array"=[]} ("Images"), "Image Sum"=w57, "Image Array"=w54) -> (w88:cluster{"Image Sum":T5, "Image Array":T5[]})
      n18 = call "AlliGator Phasor Frequency.vi"() -> ("Phasor Frequency"=w42:dbl[unit])
      n19 = Array Size(array=w61) -> (size(s)=w60:i32)
      n20 = Merge Errors(w63, w94, w90, w35) -> (w93:errorcluster)
      n21 = Array Size(array=w54) -> (size(s)=w87:i32)
      n22 = case shown="1, Default" w60 {
        selector: w60 -> [_ w145]
        tunnel: w93 -> [_ w140]
        tunnel: w92 -> [_ w189]
        tunnel: w91 -> [_ w188]
        tunnel: w89 -> [_ w187]
        tunnel: w88 -> [_ w186]
        tunnel: w87 -> [_ w185]
        tunnel: w86 -> [_ w183]
        tunnel: [w110 w182] -> w85
        tunnel: w84 -> [w116 w181]
        tunnel: [w116 w180] -> w83
        tunnel: w82 -> [w115 w179]
        tunnel: [w115 w178] -> w81
        tunnel: w80 -> [w114 w177]
        tunnel: [w114 w176] -> w79
        tunnel: w78 -> [w113 w175]
        tunnel: w77 -> [w112 w173]
        tunnel: [w112 w172] -> w76
        tunnel: w75 -> [w117 w169]
        tunnel: [w117 w168] -> w74
        tunnel: w42 -> [_ w125]
        tunnel: [_ w165] -> w73
        tunnel: w72 -> [_ w164]
        tunnel: [w113 w163] -> w71
        tunnel: [_ w162] -> w70
        tunnel: [_ w159] -> w69
        tunnel: [_ w157] -> w68
        tunnel: w66 -> [_ w156]
        tunnel: w65 -> [_ w155]
        tunnel: w64 -> [_ w154]
        tunnel: w62 -> [_ w152]
        tunnel: w61 -> [_ w150]
        tunnel: [_ w143] -> w59
        tunnel: w51 -> [_ w129]
        tunnel: w36 -> [_ w126]
        tunnel: w37 -> [_ w124]
        frame 0 {
          n23 = One Button Dialog(message="All ROIs Phasor Analysis: no ROI defined!") -> ()  [unwired: 1 in, 1 out]
          n24 = xnode "Error Ring"() -> ("error out"=w110:errorcluster)
        }
        frame 1, Default {
          n25 = call "AlliGator Get Decay Time Axis v2.vi"("Number of Gates"=w185) -> ("t Array"=w184:dbl[unit][])  [unwired: 14 in]
          n26 = call "Embedded Progress Bar Q.vi"("Progress Bar Queue Name"="AlliGator Progress Bar Q") -> ("Progress Bar Queue"=w132:refnum<queue>)  [unwired: 6 in]
          n27 = call "AlliGator Get-Set Decay Preprocessing Parameters.vi"("Get (F)/Set"=FALSE, "Error In"=w140) -> ("Error Out"=w138:errorcluster, "Decay Preprocessing Parameters out"=w134:T38)  [unwired: 8 in]
          n28 = call "Send Embedded Progress Bar Update.vi"("Max Iterations N"=w145, "Current Iteration i (i or -1: standard or || iteration; 0 or -2: first standard or || iteration)"=-2 ("Current Iteration i (-1: || iteration, -2: first || iteration)"), "Progress Bar Queue in"=w132) -> ("Error Out"=w148:errorcluster, "Progress Bar Queue out"=w149:refnum<queue>)  [unwired: 7 in]
          n29 = node(w184) -> (w153:dbl[])
          n30 = for {
            tunnel: w150 -> [w285] mode=indexing
            tunnel: w189 -> [w284]
            tunnel: w188 -> [w283]
            tunnel: w186 -> [w282]
            tunnel: w187 -> [w281]
            tunnel: [w256] -> w151
            tunnel: w153 -> [w268]
            tunnel: w183 -> [w269]
            tunnel: [w270] -> w171 mode=indexing if=w248
            tunnel: w125 -> [w280]
            tunnel: [w278] -> w141 mode=indexing if=w248
            tunnel: [w279] -> w161 mode=indexing if=w248
            tunnel: [w247] -> w174
            tunnel: [w277] -> w170 mode=indexing if=w248
            tunnel: [w276] -> w143 mode=indexing if=w248
            tunnel: [w267] -> w167
            tunnel: [w275] -> w166
            tunnel: [w274] -> w159 mode=indexing if=w263
            tunnel: w137 -> [w253]
            tunnel: [w266] -> w157
            tunnel: w156 -> [w273]
            tunnel: w155 -> [w272]
            tunnel: w154 -> [w271]
            tunnel: w152 -> [w265]
            tunnel: w145 -> [w264]
            tunnel: w148 -> [w260]
            tunnel: [w258] -> w146
            tunnel: w149 -> [w261]
            tunnel: [w259] -> w147
            tunnel: [FALSE ("Abort?")] -> w142
            tunnel: [w252] -> w139 mode=indexing
            tunnel: w134 -> [w255]
            tunnel: w129 -> [w251]
            tunnel: [w250] -> w128 mode=indexing if=w248
            tunnel: w126 -> [w245]
            tunnel: [w249] -> w127 mode=indexing if=w248
            tunnel: w124 -> [w246]
            tunnel: [w244] -> w123 mode=indexing
            tunnel: [w243] -> w122 mode=indexing
            i -> [w247]
            n31 = global read "AlliGator Abort.vi" "Abort?"() -> (w256:bool)
            n32 = call "Send Embedded Progress Bar Update.vi"("Error In"=w260, "Current Iteration i (i or -1: standard or || iteration; 0 or -2: first standard or || iteration)"=-1 ("Current Iteration i (-1: || iteration, -2: first || iteration)"), "Progress Bar Queue in"=w261) -> ("Error Out"=w258:errorcluster, "Progress Bar Queue out"=w259:refnum<queue>)  [unwired: 7 in]
            n33 = case shown="False" w256 {
              tunnel: w285 -> [w337 _]
              tunnel: w284 -> [w336 _]
              tunnel: w283 -> [w335 _]
              tunnel: w282 -> [w334 _]
              tunnel: w281 -> [w333 _]
              tunnel: w253 -> [w332 _]
              tunnel: w280 -> [w299 _]
              tunnel: [w292 _] -> w279
              tunnel: [w293 _] -> w278
              tunnel: [w327 _] -> w277
              tunnel: [w326 _] -> w276
              tunnel: [w306 _] -> w275
              tunnel: [w325 _] -> w274
              tunnel: [w323 _] -> w248
              tunnel: w273 -> [w322 _]
              tunnel: w272 -> [w321 _]
              tunnel: w271 -> [w320 _]
              tunnel: [w319 _] -> w270
              tunnel: w269 -> [w316 _]
              tunnel: w268 -> [w315 _]
              tunnel: [w298 _] -> w267
              tunnel: [w310 _] -> w266
              tunnel: w265 -> [w294 _]
              tunnel: w264 -> [w309 _]
              tunnel: w247 -> [w287 _]
              tunnel: [w308 _] -> w262
              tunnel: [w305 _] -> w252
              tunnel: w255 -> [w307 _]
              tunnel: w251 -> [w303 _]
              tunnel: [w301 _] -> w250
              tunnel: [w291 _] -> w249
              tunnel: w246 -> [w290 _]
              tunnel: w245 -> [w289 _]
              tunnel: [w288 _] -> w244
              tunnel: [w286 _] -> w243
              frame False {
                # "needed to allow pixel-to-pixel calibration\n(includes NaN + NaN i phasors)"
                n34 = Unbundle By Name(w337) -> ("ROI Descriptor"=w318:T7, "ROI Name"=w325:string)
                n35 = call "Keep String in Array.vi"("Current Index"=w287, "Number of Elements"=w309) -> ("Keep String"=w308:bool)  [unwired: 9 in]
                n36 = call "AlliGator Compute ROI Decay.vi"("Pixel Threshold High"=w336, "Loop ID"=w287, "Pixel Threshold Low"=w335, "error in (no error)"=w332, "Decay Peak  Constraints"=w333, "ROI Descriptor"=w318, "Images"=w334) -> ("error out"=w304:errorcluster, "# Valid Pixels"=w286:i32, "ROI Center"=w317:cluster{"X":i32, "Y":i32}, "Decay Points"=w314:dbl[])  [unwired: 1 out]
                n37 = Bundle(w315, "Decay Points"=w314) -> (w313:cluster{dbl[], "Decay Points":dbl[]})  [unwired: 1 in]
                n38 = call "AlliGator Preprocess Decay v3.vi"("Decay Preprocessing Parameters"=w307, "Error In"=w304, "Time-Gated Reference Decay"=w316, "# Pixels"=w286, "Decay (in)"=w313) -> ("Error Out"=w311:errorcluster, "Decay (out)"=w298:T44, "Decay Metadata"=w312:T9, "Message"=w310:string)  [unwired: 3 in]
                n39 = call "Phasor Compute Phasor from Decay v2.vi"("Error In"=w311, "Phasor Frequency"=w299, "Time-Gated Decay"=w298) -> ("Error Out"=w288:errorcluster, "s"=w330:dbl, "g"=w331:dbl)  [unwired: 5 in, 1 out]
                n40 = Bundle By Name(cluster=w312, "ROI Center"=w317, "ROI Descriptor"=w318) -> (w319:T9)
                n41 = Bundle By Name(cluster=T1 {"g"=0.0, "s"=0.0} ("Phasor"), "g"=w331, "s"=w330) -> (w328:T1)
                n42 = call "AlliGator Select Phasor Calibration v3.vi"("Calibration Map MD5 Digest"=w303, "Current Data Set (-1: single)"=w294, "ROI Center (Default: undefined)"=w317, "Error In"=w288, "Phasor Calibration Map"=w320, "Calibration Phasor Series"=w321, "Calibration Phasor"=w322) -> ("Error Out"=w300:errorcluster, "Calibration Phasor"=w301:T15)  [unwired: 1 in, 2 out]
                n43 = call "Clear Error.vi"("Error In"=w300) -> ("no Error Out"=w295:errorcluster)  [unwired: 8 in]
                n44 = Unbundle By Name(w295) -> ("status"=w324:bool)
                n45 = call "Phasor Compute Standard Deviation (Poisson).vi"("Time-Gated Decay"=w298, "Phasor SDV Options in"=w289, "Phasor Frequency"=w299, "Error In"=w295, "Calibration Phasor (m, phi)"=w301) -> ("(Mean) Phasor (g, s)"=w292:T1, "Phasor SDV (g, s)"=w291:T1, "Calibrated (Mean) Phasor (g, s)"=w297:T1)  [unwired: 4 in, 4 out]
                n46 = call "Phasor Calibration v3.vi"("Compute Lifetimes? (F)"=TRUE ("Init?"), "Error In"=w295, "Phasor Frequency"=w299, "Calibration Phasor"=w301, "Measured Phasor"=w328) -> ("Error Out"=w305:errorcluster, "Calibrated Phase Lifetime"=w306:dbl[unit], "Calibrated Phasor"=w296:T1)  [unwired: 1 in, 3 out]
                n47 = Not(x=w324) -> (.not. x?=w323:bool)
                n48 = Select(t=w297, s=w290, f=w296) -> (s? t:f=w293:T1)
                n49 = Unbundle By Name(w293) -> ("g"=w327:dbl, "s"=w326:dbl)
              }
              frame True {
              }
            }
            n50 = Compound Arithmetic op=AND(w248, w262) -> (w263:bool)
          }
          n51 = flat-sequence {
            tunnel: w125 -> [w193]
            tunnel: w138 -> [w191]
            tunnel: [w190] -> w137
            frame #0 {
              (unwired) TRUE ("want seconds? (F)")
              n52 = node(w193) -> (w192:dbl)
              n53 = call "Get Notebook Queue.vi"() -> ("Notebook Queue"=w194:refnum<queue>)  [unwired: 9 in]
              n54 = call "Current Date & Time String (High Precision).vi"() -> ("time string"=w198:string, "date string"=w197:string)  [unwired: 8 in, 2 out]
              n55 = Format Into String(format string="All ROIs Phasor Analysis (non-interactive) Started on %s at %s\nf = %#g MHz", error in=w191, w197, w198, w192) -> (resulting string=w199:string, error out=w200:errorcluster)  [unwired: 1 in]
              n56 = call "Message Style.vi"() -> ("Message Formatting"=w196:T45)
              n57 = call "Send Message to Notebook.vi"("Text Formatting"=w196, "Error In"=w200, "Message"=w199, "Notebook Queue"=w194) -> ("Error Out"=w190:errorcluster)  [unwired: 4 in, 1 out]
            }
          }
          n58 = global write "AlliGator Abort.vi" "Abort?"(w142) -> ()
          n59 = Empty Array?(array=w141) -> (empty?=w158:bool)
          n60 = call "Send Embedded Progress Bar Update.vi"("Stop Progress Bar (F)"=TRUE ("Hide Progress Bar (F)"), "Error In"=w146, "Progress Bar Queue in"=w147) -> ("Error Out"=w144:errorcluster)  [unwired: 7 in, 1 out]
          n61 = Compound Arithmetic op=OR(w158, w151) -> (w160:bool)
          n62 = Merge Errors(w139) -> (w136:errorcluster)
          n63 = case shown="False" w160 {
            tunnel: [w204 w225] -> w182
            tunnel: w181 -> [_ w234]
            tunnel: [w223 w234] -> w180
            tunnel: w179 -> [_ w228]
            tunnel: [w206 w228] -> w178
            tunnel: w177 -> [w217 w233]
            tunnel: [w216 w233] -> w176
            tunnel: w175 -> [_ w232]
            tunnel: [w219 w232] -> w163
            tunnel: w141 -> [w222 _]
            tunnel: w161 -> [w209 _]
            tunnel: w174 -> [w210 _]
            tunnel: w173 -> [_ w231]
            tunnel: [w211 w231] -> w172
            tunnel: w171 -> [w212 _]
            tunnel: w170 -> [w221 _]
            tunnel: w143 -> [w220 _]
            tunnel: w169 -> [_ w230]
            tunnel: [w218 w230] -> w168
            tunnel: w167 -> [w218 _]
            tunnel: w125 -> [w214 _]
            tunnel: w166 -> [w208 _]
            tunnel: [w208 dbl[unit] nan ("Calibrated Lifetime")] -> w165
            tunnel: w164 -> [w207 _]
            tunnel: [w206 w228] -> w162
            tunnel: w151 -> [_ w227]
            tunnel: w144 -> [_ _]
            tunnel: w136 -> [w205 _]
            tunnel: w128 -> [w203 _]
            tunnel: w126 -> [w202 _]
            tunnel: w127 -> [w201 _]
            tunnel: w123 -> [_ _]
            tunnel: w122 -> [_ _]
            frame False {
              n64 = call "Clear Error.vi"("Error In"=w205) -> ("no Error Out"=w204:errorcluster)  [unwired: 8 in]
              n65 = Bundle By Name(cluster=T8 {"Phasor Plot Name"="", "Raw Phasor Plot"=[], "Phasor Frequency"=160000000.0, "[Decay Metadata]"=[], "Raw Phasor Plot SDV"=[], "Phasor SDV Options"={"Compute Estimated SDV"=FALSE, "# Replicas"=100, "Use Estimated Average Phasor"=FALSE}, "[Calibration Phasor]"=[]} ("array"), "Phasor Frequency"=w214, "Raw Phasor Plot"=w209, "[Decay Metadata]"=w212, "Phasor Plot Name"=w207, "Raw Phasor Plot SDV"=w201, "Phasor SDV Options"=w202, "[Calibration Phasor]"=w203) -> (w213:T8)
              n66 = Bundle(w221, w220) -> (w219:cluster{dbl[], dbl[]})  [unwired: 1 in]
              n67 = Index Array(array=w209, index=w210) -> (element=w223:T1)
              n68 = Index Array(array=w222, index=w210) -> (element=w206:T1)
              n69 = Index Array(array=w212, index=w210) -> (element=w211:T9)
              n70 = Build Array (concatenate)(w217, w213) -> (w216:T8[])
            }
            frame True {
              n71 = xnode "Error Ring"() -> ("error out"=w226:errorcluster)
              n72 = xnode "Error Ring"() -> ("error out"=w224:errorcluster)
              n73 = Select(t=w226, s=w227, f=w224) -> (s? t:f=w225:errorcluster)
            }
          }
        }
      }
      n74 = in-place-cluster #2("Current Dataset Images 1.SGL Image Sum"=w41, "Current Dataset Images 1.SGL Gate Images"=w40, "Current Dataset Images 2.SGL Image Sum"=w39, "Current Dataset Images 2.SGL Gate Images"=w38, "Reference Decay"=w86, "ROI Decay"=w74, "Calibration Phasor"=w66, "Calibration Phasor Series"=w65, "Last Raw Phasor"=w83, "Last Calibrated Phasor"=w81, "[Phasor Graph:Raw Phasor Plots]"=w79, "Phasor Graph:Phasor Plot"=w71, "Decay  Metadata"=w76, "Phasor Calibration Map"=w64, "Current Dataset"=w62, "Calibration Map MD5 Digest"=w51) -> (w33:T16)
      n75 = call "Add Line Feed to String.vi"("String"=w68) -> ("String\\n"=w67:string)  [unwired: 8 in]
    }
    n76 = in-place-dvr #1(w33) -> (→"AlliGator Internal Variables DVR":refnum<data-value>)  [unwired: 1 out]
  }
  "Calibrated Phase Lifetime" <- w20
  "Phasor Plot" <- w18
  "Calibrated Phasor" <- w17
  n77 = call "High Resolution Timing.vi"("relative seconds (NaN)"=w13, "Error In"=w4) -> ("elapsed (relative) seconds"=w12:dbl, "Error Out"=w5:errorcluster)  [unwired: 15 in, 1 out]
  n78 = Array Size(array=w3) -> (size(s)=w8:i32)
  n79 = call "Concatenate String Array.vi"("Max Number of Elements (None: -1)"=8 ("Max Number of Elements (None: 1)"), "Separator (TAB)"=", ", "String Array"=w9) -> ("Formatted String"=w10:string)  [unwired: 8 in]
  n80 = call "Current Date & Time String (High Precision).vi"("Error In"=w5) -> ("Error Out"=w2:errorcluster, "on <Date> at <Time>"=w1:string)  [unwired: 7 in, 2 out]
  n81 = case shown="1, Default" w8 {
    selector: w8 -> [_ w342]
    tunnel: w1 -> [_ w348]
    tunnel: [w338 w347] -> w14
    tunnel: w12 -> [_ w345]
    tunnel: ["No valid ROIs to process..." w344] -> w11
    tunnel: w10 -> [_ w343]
    tunnel: w6 -> [_ w341]
    tunnel: w2 -> [w338 w340]
    frame 0 {
    }
    frame 1, Default {
      n82 = Format Into String(format string="All ROIs Phasor Analysis (%d):\n%s\n%scompleted %s\nCPU: %#g s", error in=w340, w342, w343, w341, w348, w345) -> (resulting string=w344:string, error out=w347:errorcluster)  [unwired: 1 in]
    }
  }
  "error out" <- w14
  "Message" <- w11
